vi "Initialize.vi"(7 "Module Model":T1=enum."NI 9210", 8 "error in":errorcluster, 9 "Slot Settings":T2, 11 "9210 in":refnum<class "9210.lvclass">) -> (0 "error out":errorcluster, 3 "9210 out":refnum<class "9210.lvclass">)   [LabVIEW 2019, in "Modules.lvlib" / "9210.lvclass"]
uses:
  9210.lvclass
  RSI Module/Slot Settings.ctl
  C:/Users/nitest/Desktop/Git 2019/niveristand-scan-engine-module-libraries/Source/RSI Module/RSI Module.lvclass
  RSI Module/Module Models.ctl
  RSI Module/Channels.ctl
  RSI Module/Channel Type.ctl
  9210.lvclass/9210.ctl
  RSI Module/RSI Module.lvclass
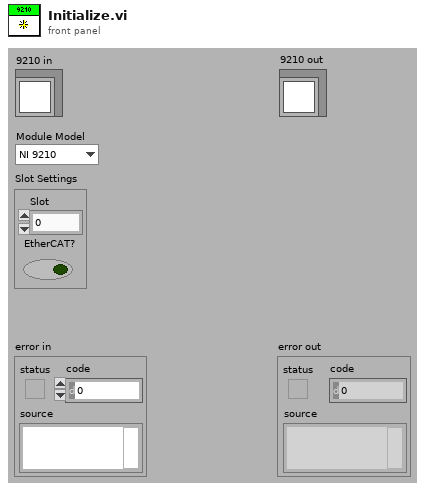
[diagram p1: front panel]
types:
  T1 = typedef "Modules.lvlib/RSI Module.lvclass/Module Models.ctl" = enum16{"Empty", "NI 9201", "NI 9203", "NI 9205", "NI 9206", "NI 9207", "NI 9208", "NI 9209", "NI 9210", "NI 9211", "NI 9212", "NI 9213", "NI 9214", "NI 9215", "NI 9216", "NI 9217", "NI 9219", "NI 9220", "NI 9221", "NI 9222", "NI 9223", "NI 9224", "NI 9225", "NI 9226", "NI 9227", "NI 9228", "NI 9229", "NI 9233", "NI 9234", "NI 9235", "NI 9236", "NI 9237", "NI 9239", "NI 9242", "NI 9244", "NI 9253", "NI 9263", "NI 9264", "NI 9265", "NI 9266", "NI 9269", "NI 9344", "NI 9350", "NI 9375", "NI 9401", "NI 9402", "NI 9403", "NI 9411", "NI 9421", "NI 9422", "NI 9423", "NI 9425", "NI 9426", "NI 9435", "NI 9436", "NI 9437", "NI 9472", "NI 9474", "NI 9475", "NI 9476", "NI 9477", "NI 9478", "NI 9481", "NI 9482", "NI 9485"}
  T2 = typedef "Modules.lvlib/RSI Module.lvclass/Slot Settings.ctl" = cluster{"Slot":u32, "EtherCAT?":bool}
  T3 = typedef "Modules.lvlib/RSI Module.lvclass/Channels.ctl" = cluster{"# Input Channels":i32, "# Output Channels":i32, "Channel Type":T4, "Units":string}
  T4 = typedef "Modules.lvlib/RSI Module.lvclass/Channel Type.ctl" = enum16{"Analog", "Digital"}
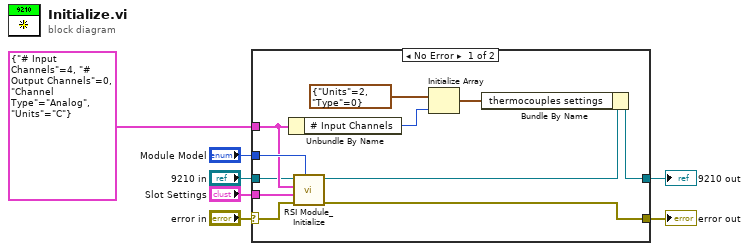
[diagram p0: block diagram]
diagram:
  n1 = case shown="No Error" "error in" {
    selector: "error in" -> [w17 w19]
    tunnel: [w16 w19] -> w6
    tunnel: [w13 _] -> w5
    tunnel: "Slot Settings" -> [w15 _]
    tunnel: "Module Model" -> [w18 _]
    tunnel: T3 {"# Input Channels"=4, "# Output Channels"=0, "Channel Type"=enum."Analog", "Units"="C"} ("Channels") -> [w12 _]
    tunnel: "9210 in" -> [w11 _]
    frame No Error {
      n2 = Unbundle By Name(w12) -> ("# Input Channels"=w10:i32)
      n3 = call "RSI Module_Initialize.vi"("Module Model"=w18, "error in (no error)"=w17, "Slot Settings"=w15, "Channels"=w12, "RSI Module in"=w11) -> ("error out"=w16:errorcluster, "RSI Module out"=w14:refnum<class "9210.lvclass">)  [unwired: 5 in]
      n4 = Initialize Array(cluster{"Units":u8, "Type":u8} {"Units"=2, "Type"=0} ("thermocouple units and type"), w10) -> (w8:cluster{"Units":u8, "Type":u8}[])
      n5 = Bundle By Name(cluster=w14, "thermocouples settings"=w8) -> (w13:refnum<class "9210.lvclass">)
    }
    frame Error {
    }
  }
  "error out" <- w6
  "9210 out" <- w5
